vi "CAENHV Get Error.vi"(8 "error in (no error)":errorcluster, 11 "handle":i32) -> (0 "error out":errorcluster, 3 "function return":string)   [LabVIEW 2009, in "CAENHVWrapper.lvlib"]
doc: "CAENHVLIB_API char *CAENHV_GetError(int handle);"
uses:
  <userlib>/CAENHVWrapper/CAENHVWrapper.lvlib
  <userlib>/CAENHVWrapper/CAENHVWrapper.dll
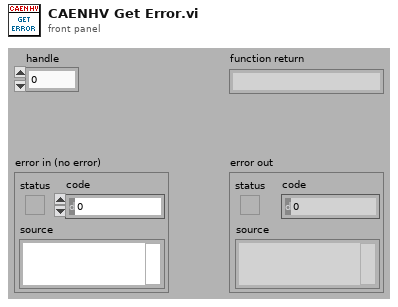
[diagram p1: front panel]
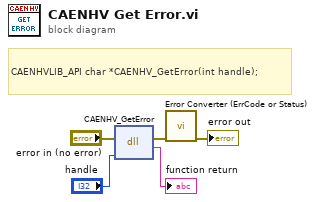
[diagram p0: block diagram]
diagram:
  # "CAENHVLIB_API char *CAENHV_GetError(int handle);"
  n1 = dll-call lib="C:/Program Files/National Instruments/LabVIEW 2009/user.lib/CAENHVWrapper/CAENHVWrapper.*" fn="CAENHV_GetError"(error in="error in (no error)", "handle"="handle") -> (error out=w2:errorcluster, →"function return":string)  [unwired: 3 in, 1 out]
  n2 = call <userlib>:"Error Converter (ErrCode or Status).vi"("error in (no error)"=w2) -> ("error out"=→"error out":errorcluster)  [unwired: 10 in]
